vi "First Char (offset).vi"(10 "offset (0)":i32, 11 "String in":string) -> (1 "First Char":string, 2 "Offset":i32)   [LabVIEW 2013, in "JSONtext support.lvlib"]
doc: "Returns first character from string."
uses:
  JSONtext support.lvlib
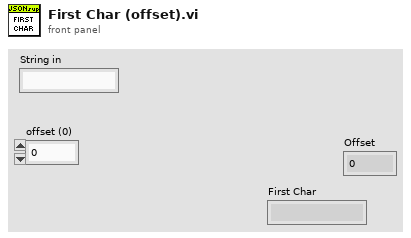
[diagram p1: front panel]
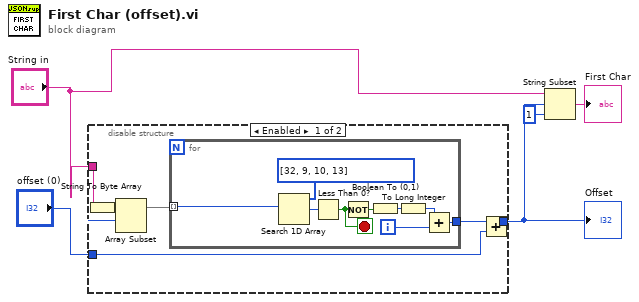
[diagram p0: block diagram]
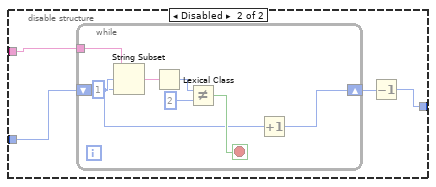
[diagram p2: hidden frame]
diagram:
  n1 = disable-structure shown="Enabled" {
    disable-tunnel: "String in" -> [w8 w23]
    disable-tunnel: "offset (0)" -> [w7 w22]
    disable-tunnel: [w6 w21] -> w1
    frame Enabled {
      n2 = String To Byte Array(string=w8) -> (unsigned byte array=w11:u8[])
      n3 = Array Subset(array=w11, index=w7) -> (w9:u8[])  [unwired: 1 in]
      n4 = for {
        tunnel: w9 -> [w19] mode=indexing
        tunnel: [w15] -> w10
        i -> [w20]
        stop <- w16 stop-if-true
        n5 = Search 1D Array(1D array=u8[] [32, 9, 10, 13], element=w19) -> (index of element=w17:i32)  [unwired: 1 in]
        n6 = Less Than 0?(x=w17) -> (x < 0?=w16:bool)
        n7 = Not(x=w16) -> (.not. x?=w13:bool)
        n8 = Boolean To (0,1)(Boolean=w13) -> (0, 1=w14:i16)
        n9 = To Long Integer(number=w14) -> (32bit integer=w12:i32)
        n10 = Add(x=w12, y=w20) -> (x+y=w15:i32)
      }
      n11 = Add(x=w10, y=w7) -> (x+y=w6:i32)
    }
    frame Disabled {
      n12 = while {
        tunnel: w23 -> [w32]
        shift-right: [w27] -> w24
        shift-left: w22 -> [w26]
        stop <- w28 stop-if-true
        n13 = String Subset(string=w32, offset (0)=w26, length (rest)=1 ("length (rest)")) -> (substring=w31:string)
        n14 = Lexical Class(1:w31) -> (0:w30:i16)
        n15 = Not Equal?(x=w30, y=i16 2) -> (x != y?=w28:bool)
        n16 = Increment(x=w26) -> (x+1=w27:i32)
      }
      n17 = Decrement(x=w24) -> (x-1=w21:i32)
    }
  }
  "Offset" <- w1
  n18 = String Subset(string="String in", offset (0)=w1, length (rest)=1 ("length (rest)")) -> (substring=→"First Char":string)
